vi "Sensor_Reference_Sensor.vi"() -> ()   [LabVIEW 2012]
doc: "This example VI demonstrates setting up a scan list and taking a reading using the advanced VIs. For more information about the different types of VIs, see the descriptions below.\n\nEven though only two types of measurements are shown, all six types can be configured in the same way. Likewise, this VI does not show every available configurable option for voltage and resistance.\n\n====================\nSetting up and performing a scan\n====================\nThe HP34970A provides commands for setting up a scan in three ways that differ in their complexity and the amount of control offered:\n\n1. Advanced:\nEvery aspect of the measurement, scan, scan list, and read is put in a different command to allow the greatest flexibility. For example, using the advanced configure VIs, you can set up a scan list consisting of different measurement types on different channels. The \"HP34970A Advanced Scan Example.vi\" demonstrates usage of these VIs.\n\n2. Medium:\nThe instrument also offers a command that wraps up configuring individual channels and the scan list. This is represented in the driver by \"HP34970A Conf EZ.vi\". This driver specifically replaces use of the advanced configure measurement VIs and configure scan list VIs. For more information, refer to the context help for the Conf EZ VI.\n\n3. Easiest:\nThe entire configuration, scan, and read are wrapped up into one command to the instrument. This is provided in this driver as the \"EZ\" VIs, which are in the Data subpalette of the HP34970A's driver palette. The \"HP34970A EZ Scan Example.vi\" demonstrates the EZ VI's usage."
uses:
  <instrlib>/Agilent 34970/Agilent 34970.lvlib
panel:
  in  "Range":T1(ring)=enum."Maximum"
  in  "NPLC":u16(ring)=2 items=[".02", ".2", "1", "2", "10", "20", "100", "200", "Minimum", "Maximum"]
  in  "DMM Channel":string
  in  "current transfer ratio":dbl[unit] caption="s"
  in  "Sample interval":dbl
  in  "Measurement done":bool
  out "standard deviation / %":dbl format="%#_3g"
  out "mean / V":dbl format="%0.2f"
  out "standard deviation / V":dbl format="%0.5f"
  out "Waveform Graph":cluster{dbl, "Interval Value (0)":dbl, dbl[]}(graph)
  out "Time / s":dbl caption="Elapsed Time (s)"
  out "Readings":string[][](array[string])
  in  "Range (Volt.)":T1(ring)=enum."Maximum"
  in  "Channel List (Volt.)":string
  in  "VISA resource name":refnum<visa-resource-name>
  # "Voltage"
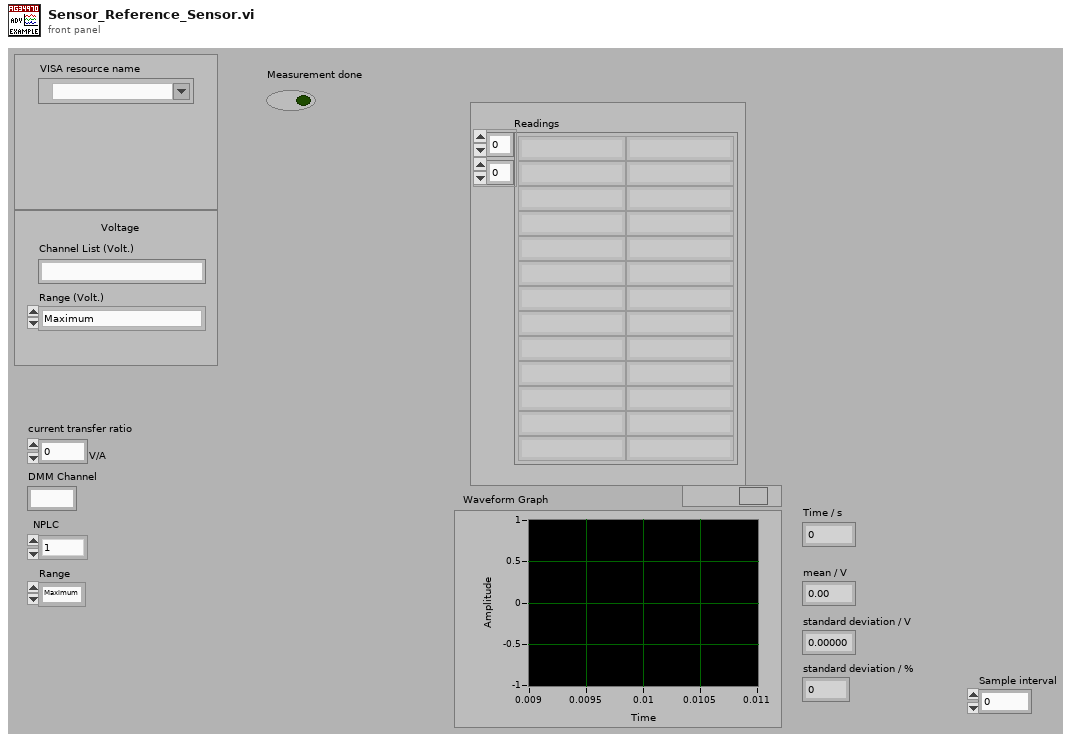
[diagram p1: front panel]
types:
  T1 = enum16{"100 mV", "1 V", "10 V", "100 V", "300 V", "Minimum", "Maximum"}
  T2 = enum16{"Remote Trigger", "Immediate Trigger", "Wait for Trigger", "Abort Scan"}
  T3 = cluster{"Include Alarm Data F:(No)":bool, "Include Channel # (F:No)":bool, "Include Time (F:No)":bool, "Include Units (F:No)":bool}
  T4 = enum16{"Manual", "Minimum", "Maximum", "Infinity"}
  T5 = enum16{"Bus", "Immediate", "External", "Alarm 1", "Alarm 2", "Alarm 3", "Alarm 4", "Timer"}
  T6 = cluster{"Timeout Value (10000)":u32, "Baud Rate (57600)":enum16{"1200", "2400", "4800", "9600", "19200", "38400", "57600", "115200"}, "Flow Control (1:XON/XOFF)":enum16{"None", "XON / XOFF", "RTS / CTS", "DTR / DSR"}}
  T7 = cluster{"Aperture Value (.4)":dbl, "Aperture (1:Minimum)":u16, "NPLC (1)":u16, "Bandwidth (3 Hz)":u16, "Input Impedance (F:Fixed)":bool, "Integration Time (F:Aperture)":bool}
  T8 = enum16{"Enable Register", "Event Register", "Operation Complete Bit"}
  T9 = cluster{"Sample interval":dbl, "Sample interval":dbl, dbl[]}
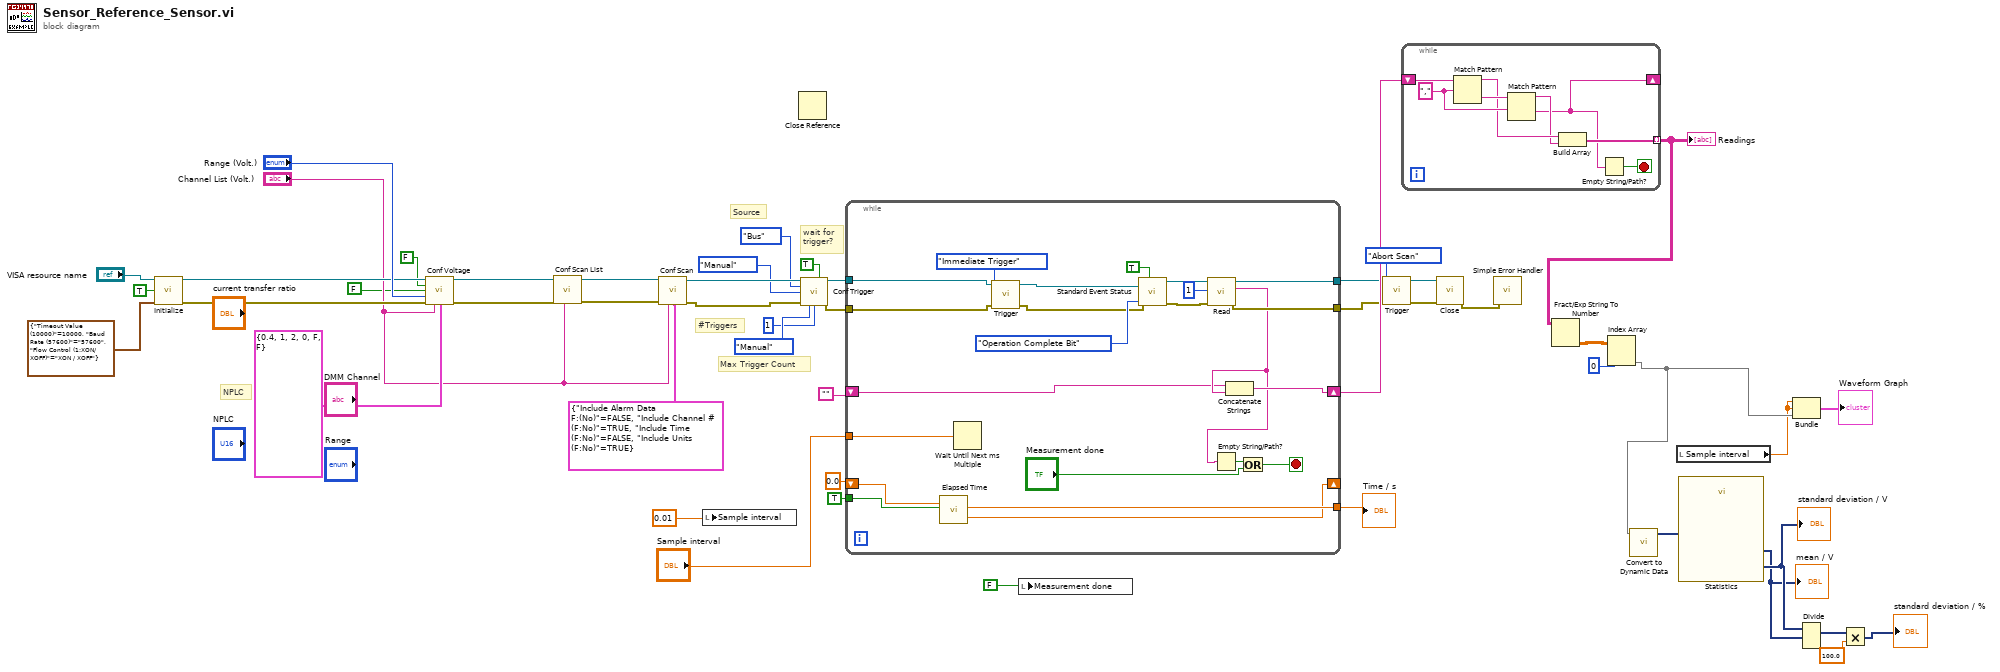
[diagram p0: block diagram]
diagram:
  # "Source"
  # "wait for \ntrigger?"
  # "Max Trigger Count"
  # "#Triggers"
  # "NPLC"
  n1 = call <instrlib>:"Initialize.vi"("VISA Resource Name"="VISA resource name", "Reset (T: Reset)"=TRUE, "Serial Port Configuration"=T6 {"Timeout Value (10000)"=10000, "Baud Rate (57600)"=enum."57600", "Flow Control (1:XON/XOFF)"=enum."XON / XOFF"}) -> ("VISA Resource Name Out"=w46:refnum<visa-resource-name>, "error out"=w30:errorcluster)  [unwired: 11 in]
  n2 = call <instrlib>:"Conf Voltage.vi"("VISA Resource Name"=w46, "AC/DC (F:DC)"=FALSE, "Autorange? (F:Off)"=FALSE, "Range (6:Max)"="Range (Volt.)", "error in (no error)"=w30, "Channel List (empty)"="Channel List (Volt.)", "Advanced Config"=T7 {"Aperture Value (.4)"=0.4, "Aperture (1:Minimum)"=1, "NPLC (1)"=2, "Bandwidth (3 Hz)"=0, "Input Impedance (F:Fixed)"=FALSE, "Integration Time (F:Aperture)"=FALSE}) -> ("VISA Resource Name Out"=w33:refnum<visa-resource-name>, "error out"=w14:errorcluster)  [unwired: 6 in, 1 out]
  n3 = call <instrlib>:"Conf Scan List.vi"("Scan List (empty)"="Channel List (Volt.)", "error in (no error)"=w14, "VISA Resource Name"=w33) -> ("error out"=w13:errorcluster, "VISA Resource Name Out"=w24:refnum<visa-resource-name>)  [unwired: 6 in, 1 out]
  n4 = call <instrlib>:"Conf Scan.vi"("VISA Resource Name"=w24, "error in (no error)"=w13, "Channel List (empty)"="Channel List (Volt.)", "Scan Fields"=T3 {"Include Alarm Data F:(No)"=FALSE, "Include Channel # (F:No)"=TRUE, "Include Time (F:No)"=FALSE, "Include Units (F:No)"=TRUE}) -> ("VISA Resource Name Out"=w28:refnum<visa-resource-name>, "error out"=w10:errorcluster)  [unwired: 9 in, 1 out]
  n5 = local write "Sample interval"(0.01 ("Samplerate")) -> ()
  n6 = Close Reference() -> ()  [unwired: 2 in, 1 out]
  n7 = call <instrlib>:"Conf Trigger.vi"("VISA Resource Name"=w28, "Wait for Trigger? (F:No)"=TRUE, "Source (1:Immediate)"=T5."Bus", "Time-Scan Interval (1:Min)"=enum16{"Manual", "Minimum", "Maximum"}."Manual", "error in (no error)"=w10, "Max Trigger Count (3:Inf)"=T4."Manual", "# Triggers (1)"=u16 1) -> ("VISA Resource Name Out"=w23:refnum<visa-resource-name>, "error out"=w22:errorcluster)  [unwired: 6 in, 1 out]
  n8 = while {
    tunnel: [w73] -> w2
    tunnel: [w72] -> w3
    tunnel: w23 -> [w65]
    tunnel: w22 -> [w71]
    shift-right: [w70] -> w45
    shift-left: "" -> [w60]
    tunnel: TRUE ("Reset") -> [w67]
    tunnel: [w66] -> w15
    shift-right: [w63] -> _
    shift-left: 0.0 ("Get Start Time (s)") -> [w64]
    tunnel: "Sample interval" -> [w59]
    stop <- w69 stop-if-true
    n9 = call "Elapsed Time"("Reset"=w67, "Set Start Time (s)"=w64) -> ("Get Start Time (s)"=w63:dbl, "Elapsed Time (s)"=w66:dbl)  [unwired: 10 in, 6 out]
    n10 = Wait Until Next ms Multiple(millisecond multiple=w59) -> ()  [unwired: 1 out]
    n11 = call <instrlib>:"Trigger.vi"("error in (no error)"=w71, "Command (0:Rem Trig)"=T2."Immediate Trigger", "VISA Resource Name"=w65) -> ("error out"=w52:errorcluster, "VISA Resource Name Out"=w53:refnum<visa-resource-name>)  [unwired: 7 in]
    n12 = call <instrlib>:"Standard Event Status.vi"("Set/Check? (F:Set)"=TRUE, "error in (no error)"=w52, "Check Parameter (0:Enable Reg)"=T8."Operation Complete Bit", "VISA Resource Name"=w53) -> ("error out"=w54:errorcluster, "VISA Resource Name Out"=w58:refnum<visa-resource-name>)  [unwired: 5 in, 1 out]
    n13 = call <instrlib>:"Read.vi"("error in (no error)"=w54, "# Channels (1)"=1 ("# Channels (0)"), "VISA Resource Name"=w58) -> ("error out"=w73:errorcluster, "Readings"=w61:string, "VISA Resource Name Out"=w72:refnum<visa-resource-name>)  [unwired: 5 in, 1 out]
    n14 = Empty String/Path?(string/path=w61) -> (empty?=w68:bool)
    n15 = Concatenate Strings(w60, w61) -> (w70:string)
    n16 = Or(x=w68, y="Measurement done") -> (x .or. y?=w69:bool)
  }
  "Time / s" <- w15
  n17 = local write "Measurement done"(FALSE ("Boolean")) -> ()
  n18 = call <instrlib>:"Trigger.vi"("error in (no error)"=w2, "Command (0:Rem Trig)"=T2."Abort Scan", "VISA Resource Name"=w3) -> ("error out"=w5:errorcluster, "VISA Resource Name Out"=w4:refnum<visa-resource-name>)  [unwired: 7 in]
  n19 = while {
    tunnel: [w76] -> w43 mode=indexing
    shift-left: w45 -> [w81]
    shift-right: [w74] -> _
    stop <- w75 stop-if-true
    w79 = "," ("regular expression")
    n20 = Match Pattern(string=w81, regular expression=w79) -> (before substring=w78:string, after substring=w80:string)  [unwired: 1 in, 2 out]
    n21 = Match Pattern(string=w80, regular expression=w79) -> (before substring=w77:string, after substring=w74:string)  [unwired: 1 in, 2 out]
    n22 = Build Array(w78, w77) -> (w76:string[])
    n23 = Empty String/Path?(string/path=w74) -> (empty?=w75:bool)
  }
  "Readings" <- w43
  n24 = call <instrlib>:"Close.vi"("VISA Resource Name"=w4, "error in (no error)"=w5) -> ("error out"=w48:errorcluster)  [unwired: 13 in]
  n25 = call <vilib>:"Simple Error Handler.vi"("error in (no error)"=w48) -> ()  [unwired: 4 in, 5 out]
  n26 = Fract/Exp String To Number(string=w43) -> (number=w42:dbl[][])  [unwired: 3 in, 1 out]
  n27 = Index Array(array=w42, index (col)=0 ("disabled index (col)")) -> (element=w34:dbl[])  [unwired: 1 in]
  n28 = call "Convert to Dynamic Data"("Array"=w34) -> ("Dynamic Data Type"=w40:dynamicdata)  [unwired: 3 in]
  n29 = local read "Sample interval"() -> (w12:dbl)
  n30 = call "Statistics"("Signals"=w40) -> ("Standard Dev"=w39:dynamicdata, "Arithmetic Mean"=w38:dynamicdata)  [unwired: 24 in, 1 out]
  "standard deviation / V" <- w39
  "mean / V" <- w38
  n31 = Bundle("Sample interval"=w12, "Sample interval"=w12, w34) -> (→"Waveform Graph":T9)  [unwired: 1 in]
  n32 = Divide(1:w38, 2:w39) -> (0:w37:dynamicdata)  [unwired: 1 in, 1 out]
  n33 = Multiply(x=w37, y=100.0) -> (x*y=→"standard deviation / %":dynamicdata)
